vi "Read SMSD Data Unit.vi"(8 "error in (no error)":errorcluster, 11 "SMSD Master in":refnum<class "SMSD Master.lvclass">) -> (0 "error out":errorcluster, 2 "IP Data Unit":refnum<class "SMSD ADU.lvclass">, 3 "SMSD Master out":refnum<class "SMSD Master.lvclass">)   [LabVIEW 2021, in "SMSD Master.lvclass"]
uses:
  SMSD Master.lvclass
  Transmission Data Unit/SMSD/SMSD ADU.lvclass
  SMSD Master.lvclass/SMSD Master.ctl
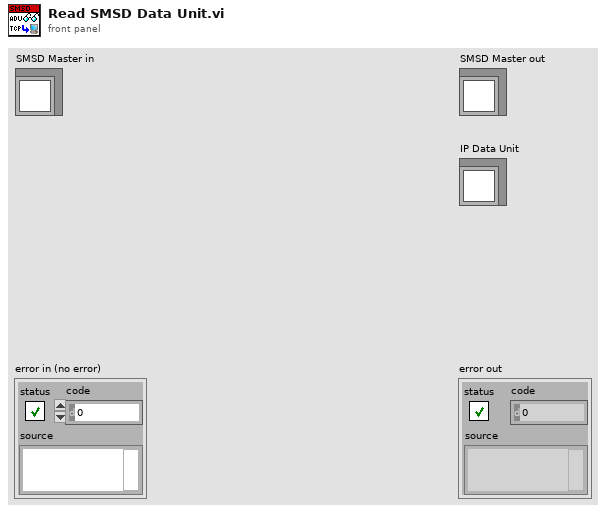
[diagram p1: front panel]
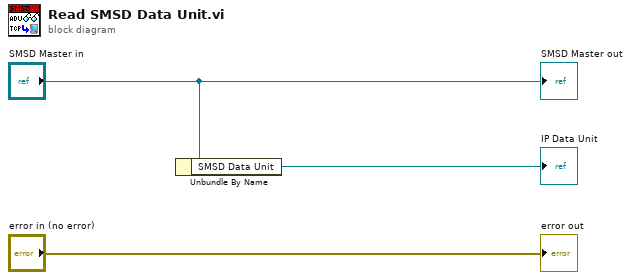
[diagram p0: block diagram]
diagram:
  n1 = Unbundle By Name("SMSD Master in") -> ("SMSD Data Unit"=→"IP Data Unit":refnum<class "SMSD ADU.lvclass">)
  "error out" <- "error in (no error)"
  "SMSD Master out" <- "SMSD Master in"
